vi "AuMT8852B EDR Test Parameter.vi"(0 "VISA session":refnum<visa-resource-name>, 1 "Test (Output power)":T2(ring), 2 "Parameter (Use low frequency)":T1, 3 "Range check? (F)":bool, 4 "Simulate? (F)":bool, 5 "error in (no error)":errorcluster, 6 "Set/Get (Set)":enum16{"Set", "Get"}(ring), 8 "Script (3)":i32=3, 10 "Integer value (0)":i32, 12 "Float value (0)":dbl format="%.3f") -> (11 "Integer value out":i32, 13 "Float value out":dbl format="%.3f", 14 "VISA session out":refnum<visa-resource-name>, 19 "error out":errorcluster)   [LabVIEW 2017]
doc: "Anritsu MT8852B Bluetooth Tester\n\nWrites or reads a single test parameter from the instrument. This VI is a tool for use by higher-level configuration functions. Not all combinations of tests and parameters are valid.\n\nINPUTS\nSet/Get - whether the parameter will be sent to or received from the instrument.\nScript - test script (1-10) containing the test being configured. Scripts 1 and 2 are read-only.\nTest - type of test to be configured.\nParameter - property of the test to be read or written.\nRange check? - whether or not this VI should reject out-of-range values.\nSimulate? - whether or not this VI should skip the instrument I/O.\nInteger value - value to be written (for integer/boolean parameters).\nFloat value - value to be written (for floating-point parameters).\n\nOUTPUTS\nInteger value out - value read from instrument (for integer/boolean parameters).\nFloat value out - value read from instrument (for floating-point parameters)."
uses:
  <instrlib>/aumt8852B/General/Utilities/MT8850 Test Parameters.ctl
  <instrlib>/aumt8852B/General/Utilities/MT8850 Frequency Units.ctl
panel:
  out "Response":string
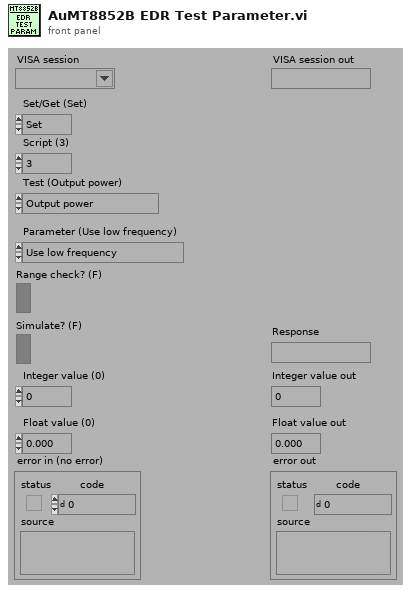
[diagram p1: front panel]
types:
  T1 = typedef "MT8850 Test Parameters.ctl" = enum16{"Use low frequency", "Use medium frequency", "Use high frequency", "Low TX frequency", "Low RX frquency", "Medium TX frequency", "Medium RX frequency", "High TX frequency", "High RX frequency", "Number of packets", "Average high limit", "Average low limit", "Peak power limit", "Max power step limit", "Min power step limit", "f1 average minimum", "f1 average maximum", "f2 maximum", "f1/f2 average maximum", "Hop selection", "Use DH1 packets", "Use DH3 packets", "Use DH5 packets", "1 slot packet drift limit", "3 slot packet drift limit", "5 slot packet drift limit", "Drift rate limit", "TX power level", "Frequency offset", "Symbol timing", "Modulation index", "BER limit", "FER limit", "Use averaging high limit", "Use averaging low limit", "Use peak power limit", "Packet type", "Test control", "Use max power step limit", "Use min power step limit", "Number of cycles", "Use f1 average maximum", "Use f1 average minimum", "Use f2 maximum", "Use f1/f2 average maximum", "Hop mode", "Maximum negative limit", "Maximum positive limit", "Use maximum negative limit", "Use maximum positive limit", "Use 1 slot packet drift limit", "Use 3 slot packet drift limit", "Use 5 slot packet drift limit", "Use drift rate limit", "Use BER limit", "Use FER limit", "Use dirty parameter table", "Use null packet drift limit", "Null packet drift limit", "Minimum power", "Power delay", "Packet count", "Payload toggle", "Output power level", "2DHX packet type", "3DHX packet type", "Number of blocks", "TX and RX low frequency", "TX and RX medium frequency", "TX and RX high frequency", "TX frequency", "RX frequency", "Threshold bit count", "Total test bit count", "Number of bits", "PDPSK to PGFSK lower limit", "PDPSK to PGFSK upper limit", "Initial frequency error upper limit", "Initial frequency error lower limit", "Frequency error upper limit", "Frequency error lower limit", "Block frequency error upper limit", "Block frequency error lower limit", "2Mbs RMS DEVM limit", "3Mbs RMS DEVM limit", "2Mbs Peak DEVM limit", "3Mbs Peak DEVM limit", "2Mbs 99% packets DEVM limit", "3Mbs 99% packets DEVM limit", "Percentage of no error packets limit", "Threshold error limit", "Total test error limit"}
  T2 = enum16{"Output power", "Power control", "Modulation characteristics", "Initial carrier", "Carrier drift", "Single slot sensitivity", "Multiple slot sensitivity", "Maximum input power", "EDR Relative transmit power", "EDR Carrier frequency and stability", "EDR Differential phase encoding", "EDR Sensitivity", "EDR BER floor sensitivity", "EDR Maximum input power"}
  T3 = typedef "MT8850 Frequency Units.ctl" = enum16{"Channel", "Hz", "kHz", "MHz", "GHz"}
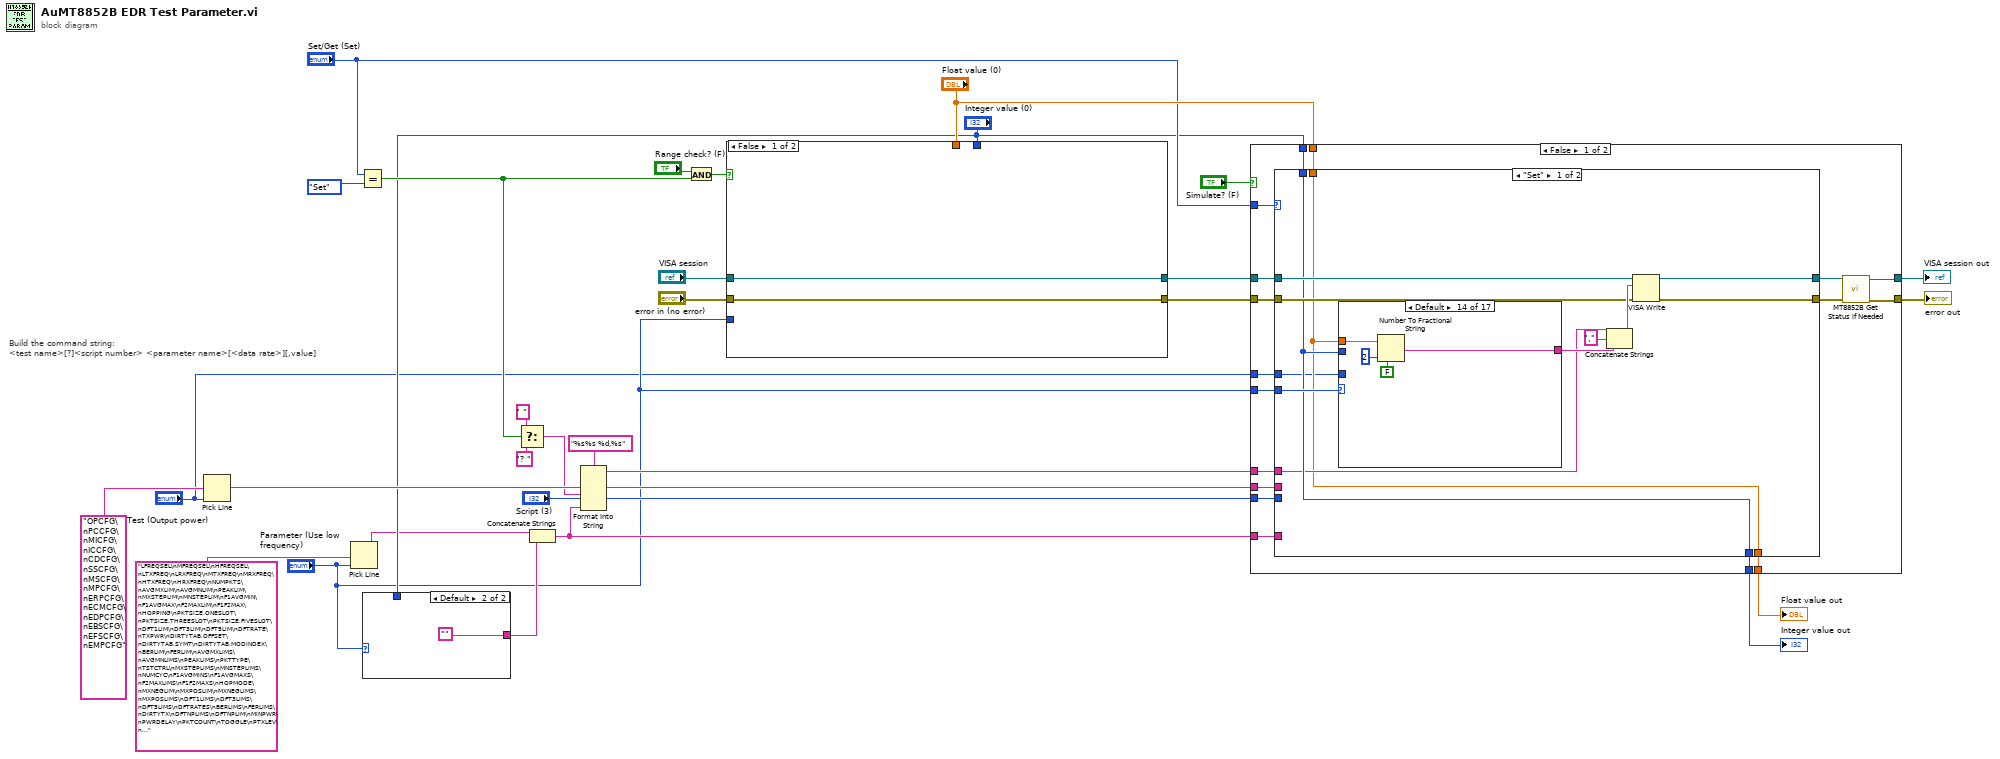
[diagram p0: block diagram]
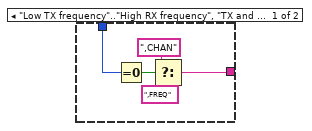
[diagram p2: hidden frame]
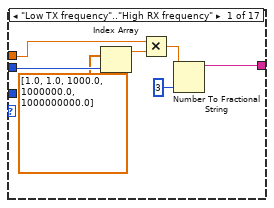
[diagram p3: hidden frame]
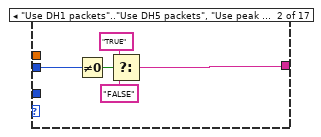
[diagram p4: hidden frame]
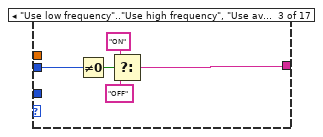
[diagram p5: hidden frame]
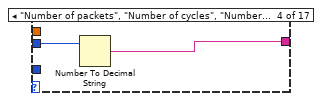
[diagram p6: hidden frame]
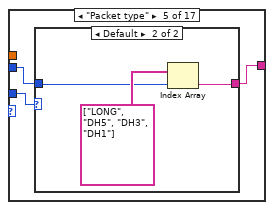
[diagram p7: hidden frame]
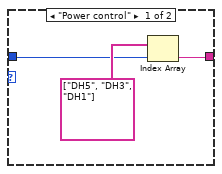
[diagram p8: hidden frame]
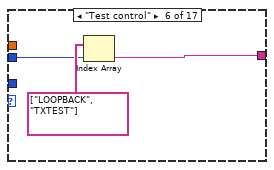
[diagram p9: hidden frame]
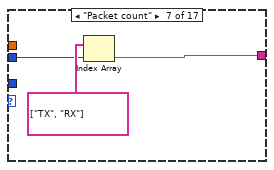
[diagram p10: hidden frame]
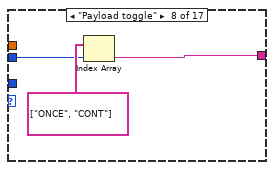
[diagram p11: hidden frame]
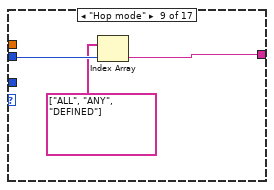
[diagram p12: hidden frame]
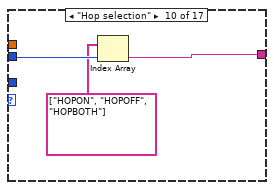
[diagram p13: hidden frame]
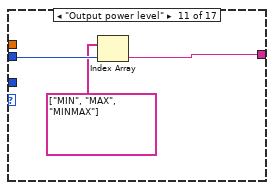
[diagram p14: hidden frame]
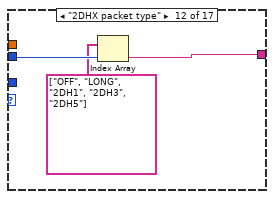
[diagram p15: hidden frame]
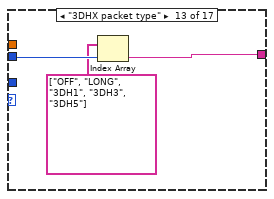
[diagram p16: hidden frame]
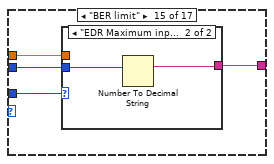
[diagram p17: hidden frame]
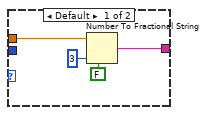
[diagram p18: hidden frame]
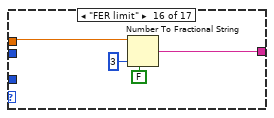
[diagram p19: hidden frame]
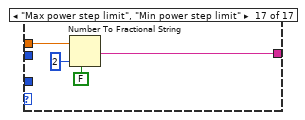
[diagram p20: hidden frame]
diagram:
  # "Build the command string:\n<test name>[?]<script number> <parameter name>[<data rate>][,value]"
  n1 = Pick Line(multi-line string="OPCFG\nPCCFG\nMICFG\nICCFG\nCDCFG\nSSCFG\nMSCFG\nMPCFG\nERPCFG\nECMCFG\nEDPCFG\nEBSCFG\nEFSCFG\nEMPCFG", line index="Test (Output power)") -> (output string=w12:string)  [unwired: 1 in]
  n2 = Pick Line(multi-line string="LFREQSEL\nMFREQSEL\nHFREQSEL\nLTXFREQ\nLRXFREQ\nMTXFREQ\nMRXFREQ\nHTXFREQ\nHRXFREQ\nNUMPKTS\nAVGMXLIM\nAVGMNLIM\nPEAKLIM\nMXSTEPLIM\nMNSTEPLIM\nF1AVGMIN\nF1AVGMAX\nF2MAXLIM\nF1F2MAX\nHOPPING\nPKTSIZE,ONESLOT\nPKTSIZE,THREESLOT\nPKTSIZE,FIVESLOT\nDFT1LIM\nDFT3LIM\nDFT5LIM\nDFTRATE\nTXPWR\nDIRTYTAB,OFFSET\nDIRTYTAB,SYMT\nDIRTYTAB,MODINDEX\nBERLIM\nFERLIM\nAVGMXLIMS\nAVGMNLIMS\nPEAKLIMS\nPKTTYPE\nTSTCTRL\nMXSTEPLIMS\nMNSTEPLIMS\nNUMCYC\nF1AVGMINS\nF1AVGMAXS\nF2MAXLIMS\nF1F2MAXS\nHOPMODE\nMXNEGLIM\nMXPOSLIM\nMXNEGLIMS\nMXPOSLIMS\nDFT1LIMS\nDFT3LIMS\nDFT5LIMS\nDFTRATES\nBERLIMS\nFERLIMS\nDIRTYTX\nDFTNPLIMS\nDFTNPLIM\nMINPWR\nPWRDELAY\nPKTCOUNT\nTOGGLE\nPTXLEV\nDHXPKT,2\nDHXPKT,3\nNUMBLKS\nLFREQ\nMFREQ\nHFREQ\nTXFREQ\nRXFREQ\nTHBITCNT\nTTBITCNT\nNUMBITS\nPDIFFLL\nPDIFFLH\nINITFRQLH\nINITFRQLL\nFREQERLH\nFREQERLL\nBLKFRQLH\nBLKFRQLL\nLRMSDEVM\nHRMSDEVM\nLPKDEVM\nHPKDEVM\nLPCTDEVM\nHPCTDEVM\nPCTPKT\nTHERR\nTTERR\n", line index="Parameter (Use low frequency)") -> (output string=w6:string)  [unwired: 1 in]
  n3 = Equal?(x="Set/Get (Set)", y=enum16{"Set", "Get"}."Set") -> (x = y?=w22:bool)
  n4 = case shown="Default" "Parameter (Use low frequency)" {
    tunnel: "Integer value (0)" -> [w35 _]
    tunnel: [w31 ""] -> w5
    frame "Low TX frequency".."High RX frequency", "TX and RX low frequency".."RX frequency" {
      n5 = Equal To 0?(x=w35) -> (x = 0?=w34:bool)
      n6 = Select(t=",CHAN" ("Substring"), s=w34, f=",FREQ" ("Substring")) -> (s? t:f=w31:string)
    }
    frame Default {
    }
  }
  n7 = Select(t=" ", s=w22, f="? ") -> (s? t:f=w11:string)
  n8 = Concatenate Strings(w6, w5) -> (w7:string)
  n9 = Format Into String(format string="%s%s %d,%s" ("Format String"), w12, w11, "Script (3)", w7) -> (resulting string=w4:string)  [unwired: 2 in, 1 out]
  n10 = And(x="Range check? (F)", y=w22) -> (x .and. y?=w24:bool)
  n11 = case shown="False" w24 {
    tunnel: "Parameter (Use low frequency)" -> [_ w45]
    tunnel: "Integer value (0)" -> [_ w44]
    tunnel: "Float value (0)" -> [_ w43]
    tunnel: "VISA session" -> [w38 w42]
    tunnel: "error in (no error)" -> [w37 w41]
    tunnel: [w38 w40] -> w19
    tunnel: [w37 w39] -> w18
    frame False {
    }
    frame True {
      n12 = case shown="\"Number of packets\", \"Number of cycles\"" w45 {
        tunnel: w44 -> [_ w50 w75 w83 _ _ w105 w111 _ _ _ _ _ _ _ _ _ _]
        tunnel: w43 -> [_ w48 _ _ w92 w100 _ _ w119 w127 w135 w143 w151 w159 w167 w175 w183 w191]
        tunnel: w42 -> [w47 w56 w72 w80 w88 w96 w103 w113 w121 w129 w137 w145 w153 w161 w169 w177 w185 w193]
        tunnel: w41 -> [w46 w55 w71 w79 w87 w95 w104 w112 w120 w128 w136 w144 w152 w160 w168 w176 w184 w192]
        tunnel: [w47 w58 w70 w78 w86 w94 w102 w110 w118 w126 w134 w142 w150 w158 w166 w174 w182 w190] -> w40
        tunnel: [w46 w57 w69 w77 w85 w93 w101 w109 w117 w125 w133 w141 w149 w157 w165 w173 w181 w189] -> w39
        frame Default {
        }
        frame "Low TX frequency".."High RX frequency", "TX and RX low frequency".."RX frequency" {
          n13 = Type Cast(type=MT8850_Frequency_Units."MHz" ("Frequency units (MHz)"), x=w50) -> (*(type *) &x=w51:T3)
          n14 = case shown="\"Channel\"" w51 {
            tunnel: [78.0 2480000000.0 2480000.0 2480.0 2.48] -> w54
            tunnel: [0.0 2402000000.0 2402000.0 2402.0 2.402] -> w53
            frame "Channel" {
            }
            frame "Hz" {
            }
            frame "kHz" {
            }
            frame "MHz" {
            }
            frame "GHz" {
            }
          }
          n15 = call <instrlib>:"AuMT8852B Check Float Range.vi"("Value (0)"=w48, "Check IVI flag first? (T)"=FALSE, "error in (no error)"=w55, "Lower limit (-1)"=w53, "Upper limit (1)"=w54, "VISA session"=w56) -> ("error out"=w57:errorcluster, "VISA session out"=w58:refnum<visa-resource-name>)  [unwired: 4 in]
        }
        frame "Number of packets", "Number of cycles" {
          n16 = call <instrlib>:"AuMT8852B Check Integer Range.vi"("Value (0)"=w75, "Check IVI flag first? (T)"=FALSE, "error in (no error)"=w71, "Lower limit (-1)"=1, "Upper limit (1)"=10000, "VISA session"=w72) -> ("error out"=w69:errorcluster, "VISA session out"=w70:refnum<visa-resource-name>)  [unwired: 4 in]
        }
        frame "Number of blocks" {
          n17 = call <instrlib>:"AuMT8852B Check Integer Range.vi"("Value (0)"=w83, "Check IVI flag first? (T)"=FALSE, "error in (no error)"=w79, "Lower limit (-1)"=1, "Upper limit (1)"=500, "VISA session"=w80) -> ("error out"=w77:errorcluster, "VISA session out"=w78:refnum<visa-resource-name>)  [unwired: 4 in]
        }
        frame "Average high limit".."Peak power limit" {
          n18 = call <instrlib>:"AuMT8852B Check Float Range.vi"("Value (0)"=w92, "Check IVI flag first? (T)"=FALSE, "error in (no error)"=w87, "Lower limit (-1)"=-80.0, "Upper limit (1)"=30.0, "VISA session"=w88) -> ("error out"=w85:errorcluster, "VISA session out"=w86:refnum<visa-resource-name>)  [unwired: 4 in]
        }
        frame "Threshold bit count".."Number of bits" {
          n19 = call <instrlib>:"AuMT8852B Check Float Range.vi"("Value (0)"=w100, "Check IVI flag first? (T)"=FALSE, "error in (no error)"=w95, "Lower limit (-1)"=1.0, "Upper limit (1)"=999.0, "VISA session"=w96) -> ("error out"=w93:errorcluster, "VISA session out"=w94:refnum<visa-resource-name>)  [unwired: 4 in]
        }
        frame "Threshold error limit", "Total test error limit" {
          n20 = call <instrlib>:"AuMT8852B Check Integer Range.vi"("Value (0)"=w105, "Check IVI flag first? (T)"=FALSE, "error in (no error)"=w104, "Lower limit (-1)"=1, "Upper limit (1)"=999, "VISA session"=w103) -> ("error out"=w101:errorcluster, "VISA session out"=w102:refnum<visa-resource-name>)  [unwired: 4 in]
        }
        frame "Max power step limit", "Min power step limit" {
          n21 = call <instrlib>:"AuMT8852B Check Integer Range.vi"("Value (0)"=w111, "Check IVI flag first? (T)"=FALSE, "error in (no error)"=w112, "Lower limit (-1)"=1, "Upper limit (1)"=10, "VISA session"=w113) -> ("error out"=w109:errorcluster, "VISA session out"=w110:refnum<visa-resource-name>)  [unwired: 4 in]
        }
        frame "Frequency offset" {
          n22 = call <instrlib>:"AuMT8852B Check Float Range.vi"("Value (0)"=w119, "Check IVI flag first? (T)"=FALSE, "error in (no error)"=w120, "Lower limit (-1)"=-75000.0, "Upper limit (1)"=75000.0, "VISA session"=w121) -> ("error out"=w117:errorcluster, "VISA session out"=w118:refnum<visa-resource-name>)  [unwired: 4 in]
        }
        frame "Symbol timing" {
          n23 = call <instrlib>:"AuMT8852B Check Float Range.vi"("Value (0)"=w127, "Check IVI flag first? (T)"=FALSE, "error in (no error)"=w128, "Lower limit (-1)"=-20.0, "Upper limit (1)"=20.0, "VISA session"=w129) -> ("error out"=w125:errorcluster, "VISA session out"=w126:refnum<visa-resource-name>)  [unwired: 4 in]
        }
        frame "Modulation index" {
          n24 = call <instrlib>:"AuMT8852B Check Float Range.vi"("Value (0)"=w135, "Check IVI flag first? (T)"=FALSE, "error in (no error)"=w136, "Lower limit (-1)"=0.25, "Upper limit (1)"=0.38, "VISA session"=w137) -> ("error out"=w133:errorcluster, "VISA session out"=w134:refnum<visa-resource-name>)  [unwired: 4 in]
        }
        frame "Minimum power" {
          n25 = call <instrlib>:"AuMT8852B Check Float Range.vi"("Value (0)"=w143, "Check IVI flag first? (T)"=FALSE, "error in (no error)"=w144, "Lower limit (-1)"=-40.0, "Upper limit (1)"=0.0, "VISA session"=w145) -> ("error out"=w141:errorcluster, "VISA session out"=w142:refnum<visa-resource-name>)  [unwired: 4 in]
        }
        frame "Power delay" {
          n26 = call <instrlib>:"AuMT8852B Check Float Range.vi"("Value (0)"=w151, "Check IVI flag first? (T)"=FALSE, "error in (no error)"=w152, "Lower limit (-1)"=0.1, "Upper limit (1)"=100.0, "VISA session"=w153) -> ("error out"=w149:errorcluster, "VISA session out"=w150:refnum<visa-resource-name>)  [unwired: 4 in]
        }
        frame "PDPSK to PGFSK lower limit" {
          n27 = call <instrlib>:"AuMT8852B Check Float Range.vi"("Value (0)"=w159, "Check IVI flag first? (T)"=FALSE, "error in (no error)"=w160, "Lower limit (-1)"=0.0, "Upper limit (1)"=8.0, "VISA session"=w161) -> ("error out"=w157:errorcluster, "VISA session out"=w158:refnum<visa-resource-name>)  [unwired: 4 in]
        }
        frame "PDPSK to PGFSK upper limit" {
          n28 = call <instrlib>:"AuMT8852B Check Float Range.vi"("Value (0)"=w167, "Check IVI flag first? (T)"=FALSE, "error in (no error)"=w168, "Lower limit (-1)"=0.0, "Upper limit (1)"=4.0, "VISA session"=w169) -> ("error out"=w165:errorcluster, "VISA session out"=w166:refnum<visa-resource-name>)  [unwired: 4 in]
        }
        frame "Initial frequency error upper limit".."Block frequency error lower limit" {
          n29 = call <instrlib>:"AuMT8852B Check Float Range.vi"("Value (0)"=w175, "Check IVI flag first? (T)"=FALSE, "error in (no error)"=w176, "Lower limit (-1)"=-100000.0, "Upper limit (1)"=100000.0, "VISA session"=w177) -> ("error out"=w173:errorcluster, "VISA session out"=w174:refnum<visa-resource-name>)  [unwired: 4 in]
        }
        frame "2Mbs RMS DEVM limit".."3Mbs 99% packets DEVM limit" {
          n30 = call <instrlib>:"AuMT8852B Check Float Range.vi"("Value (0)"=w183, "Check IVI flag first? (T)"=FALSE, "error in (no error)"=w184, "Lower limit (-1)"=0.0, "Upper limit (1)"=0.1, "VISA session"=w185) -> ("error out"=w181:errorcluster, "VISA session out"=w182:refnum<visa-resource-name>)  [unwired: 4 in]
        }
        frame "Percentage of no error packets limit" {
          n31 = call <instrlib>:"AuMT8852B Check Float Range.vi"("Value (0)"=w191, "Check IVI flag first? (T)"=FALSE, "error in (no error)"=w192, "Lower limit (-1)"=1.0, "Upper limit (1)"=99.0, "VISA session"=w193) -> ("error out"=w189:errorcluster, "VISA session out"=w190:refnum<visa-resource-name>)  [unwired: 4 in]
        }
      }
    }
  }
  n32 = case shown="False" "Simulate? (F)" {
    tunnel: "Parameter (Use low frequency)" -> [w213 _]
    tunnel: "Integer value (0)" -> [w212 w395]
    tunnel: "Float value (0)" -> [w211 w394]
    tunnel: "Set/Get (Set)" -> [w210 _]
    tunnel: w4 -> [w205 _]
    tunnel: w19 -> [w209 w393]
    tunnel: w18 -> [w208 w392]
    tunnel: [w198 w393] -> w17
    tunnel: [w197 w392] -> w10
    tunnel: [w207 w395] -> w16
    tunnel: [w206 w394] -> w15
    tunnel: w12 -> [w204 _]
    tunnel: w7 -> [w203 _]
    tunnel: "Script (3)" -> [w202 _]
    tunnel: "Test (Output power)" -> [w201 _]
    frame False {
      n33 = case shown="\"Set\"" w210 {
        tunnel: w213 -> [w225 w314]
        tunnel: w212 -> [w217 w311]
        tunnel: w211 -> [w215 w310]
        tunnel: w205 -> [w216 w320]
        tunnel: w209 -> [w221 w322]
        tunnel: w208 -> [w220 w321]
        tunnel: [w219 w316] -> w200
        tunnel: [w218 w315] -> w199
        tunnel: [w217 w313] -> w207
        tunnel: [w215 w312] -> w206
        tunnel: w204 -> [_ w308]
        tunnel: w203 -> [_ w306]
        tunnel: w202 -> [_ w307]
        tunnel: w201 -> [w214 w300]
        frame "Set" {
          n34 = case shown="Default" w225 {
            tunnel: w217 -> [w232 w234 w239 w244 w247 w255 w258 w261 w265 w268 w271 w274 w277 _ w282 _ _]
            tunnel: w215 -> [w230 _ _ _ _ _ _ _ _ _ _ _ _ w281 w284 w293 w299]
            tunnel: [w226 w233 w238 w243 w246 w254 w257 w260 w264 w267 w270 w273 w276 w280 w283 w292 w298] -> w223
            tunnel: w214 -> [_ _ _ _ w245 _ _ _ _ _ _ _ _ _ w285 _ _]
            frame "Low TX frequency".."High RX frequency" {
              n35 = Index Array(array=dbl[] [1.0, 1.0, 1000.0, 1000000.0, 1000000000.0] ("Array Constant"), index=w232) -> (element=w231:dbl)
              n36 = Multiply(x=w230, y=w231) -> (x*y=w228:dbl)
              n37 = Number To Fractional String(number=w228, precision (6)=i16 3) -> (F-format string=w226:string)  [unwired: 2 in]
            }
            frame "Use DH1 packets".."Use DH5 packets", "Use peak power limit", "Use max power step limit", "Use min power step limit", "Use f1 average maximum".."Use f1/f2 average maximum", "Use maximum negative limit".."Use FER limit" {
              n38 = Not Equal To 0?(x=w234) -> (x != 0?=w237:bool)
              n39 = Select(t="TRUE", s=w237, f="FALSE") -> (s? t:f=w233:string)
            }
            frame "Use low frequency".."Use high frequency", "Use averaging high limit", "Use averaging low limit", "Use dirty parameter table", "Use null packet drift limit" {
              n40 = Not Equal To 0?(x=w239) -> (x != 0?=w242:bool)
              n41 = Select(t="ON", s=w242, f="OFF") -> (s? t:f=w238:string)
            }
            frame "Number of packets", "Number of cycles", "Number of blocks", "Threshold error limit", "Total test error limit" {
              n42 = Number To Decimal String(number=w244) -> (decimal integer string=w243:string)  [unwired: 1 in]
            }
            frame "Packet type" {
              n43 = case shown="Default" w245 {
                tunnel: w247 -> [w249 w252]
                tunnel: [w248 w251] -> w246
                frame "Power control" {
                  n44 = Index Array(array=string[] ["DH5", "DH3", "DH1"] ("Array Constant"), index=w249) -> (element=w248:string)
                }
                frame Default {
                  n45 = Index Array(array=string[] ["LONG", "DH5", "DH3", "DH1"] ("Array Constant"), index=w252) -> (element=w251:string)
                }
              }
            }
            frame "Test control" {
              n46 = Index Array(array=string[] ["LOOPBACK", "TXTEST"] ("Array Constant"), index=w255) -> (element=w254:string)
            }
            frame "Packet count" {
              n47 = Index Array(array=string[] ["TX", "RX"] ("Array Constant"), index=w258) -> (element=w257:string)
            }
            frame "Payload toggle" {
              n48 = Index Array(array=string[] ["ONCE", "CONT"] ("Array Constant"), index=w261) -> (element=w260:string)
            }
            frame "Hop mode" {
              n49 = Index Array(array=string[] ["ALL", "ANY", "DEFINED"] ("Array Constant"), index=w265) -> (element=w264:string)
            }
            frame "Hop selection" {
              n50 = Index Array(array=string[] ["HOPON", "HOPOFF", "HOPBOTH"] ("Array Constant"), index=w268) -> (element=w267:string)
            }
            frame "Output power level" {
              n51 = Index Array(array=string[] ["MIN", "MAX", "MINMAX"] ("Array Constant"), index=w271) -> (element=w270:string)
            }
            frame "2DHX packet type" {
              n52 = Index Array(array=string[] ["OFF", "LONG", "2DH1", "2DH3", "2DH5"] ("Array Constant"), index=w274) -> (element=w273:string)
            }
            frame "3DHX packet type" {
              n53 = Index Array(array=string[] ["OFF", "LONG", "3DH1", "3DH3", "3DH5"] ("Array Constant"), index=w277) -> (element=w276:string)
            }
            frame Default {
              n54 = Number To Fractional String(use system decimal point (T)=FALSE, number=w281, precision (6)=i16 2) -> (F-format string=w280:string)  [unwired: 1 in]
            }
            frame "BER limit" {
              n55 = case shown="\"EDR Maximum input power\"" w285 {
                tunnel: w284 -> [w287 _]
                tunnel: [w286 w291] -> w283
                tunnel: w282 -> [_ w290]
                frame Default {
                  n56 = Number To Fractional String(use system decimal point (T)=FALSE, number=w287, precision (6)=i16 3) -> (F-format string=w286:string)  [unwired: 1 in]
                }
                frame "EDR Maximum input power" {
                  n57 = Number To Decimal String(number=w290) -> (decimal integer string=w291:string)  [unwired: 1 in]
                }
              }
            }
            frame "FER limit" {
              n58 = Number To Fractional String(use system decimal point (T)=FALSE, number=w293, precision (6)=i16 3) -> (F-format string=w292:string)  [unwired: 1 in]
            }
            frame "Max power step limit", "Min power step limit" {
              n59 = Number To Fractional String(use system decimal point (T)=FALSE, number=w299, precision (6)=i16 2) -> (F-format string=w298:string)  [unwired: 1 in]
            }
          }
          n60 = Concatenate Strings(w216, "," ("Substring"), w223) -> (w222:string)
          n61 = VISA Write(VISA resource name=w221, write buffer=w222, error in (no error)=w220) -> (VISA resource name out=w219:refnum<visa-resource-name>, error out=w218:errorcluster)  [unwired: 1 out]
        }
        frame "Get" {
          n62 = VISA Write(VISA resource name=w322, write buffer=w320, error in (no error)=w321) -> (VISA resource name out=w319:refnum<visa-resource-name>, error out=w318:errorcluster)  [unwired: 1 out]
          n63 = Format Into String(format string="%s %d,%s,%%s" ("Format String"), w308, w307, w306) -> (resulting string=w305:string)  [unwired: 2 in, 1 out]
          n64 = VISA Read(VISA resource name=w319, byte count=u32 100 ("byte count (0)"), error in (no error)=w318) -> (VISA resource name out=w316:refnum<visa-resource-name>, read buffer=w303:string, error out=w315:errorcluster)  [unwired: 1 out]
          n65 = Match Pattern(string=w303, regular expression="\n$") -> (before substring=w301:string)  [unwired: 1 in, 3 out]
          n66 = Scan From String(format string=w305, input string=w301) -> (output 1=w304:string)  [unwired: 3 in, 3 out]
          "Response" <- w304
          n67 = case shown="\"Number of packets\", \"Number of cycles\", \"Number of blocks\", \"Threshold error limit\", \"Total test error limit\"" w314 {
            tunnel: w304 -> [w328 w331 w334 w338 w342 w346 w350 w354 w358 w362 w366 w370 w375 w385 w391]
            tunnel: [w327 w330 w333 w337 w341 w345 w349 w353 w357 w361 w365 w368 w373 w383 w386] -> w313
            tunnel: [w326 w329 w332 w336 w340 w344 w348 w352 w356 w360 w364 w369 w374 w384 w387] -> w312
            tunnel: w311 -> [_ _ _ _ _ _ _ _ _ _ _ w368 w372 w383 w386]
            tunnel: w310 -> [w326 w329 w332 w336 w340 w344 w348 w352 w356 w360 w364 _ w371 _ _]
            tunnel: w300 -> [_ _ _ _ _ _ _ _ _ _ _ _ w376 _ _]
            frame "Use low frequency".."Use high frequency", "Use DH1 packets".."Use DH5 packets", "Use averaging high limit".."Use peak power limit", "Use max power step limit", "Use min power step limit", "Use f1 average maximum".."Use f1/f2 average maximum", "Use maximum negative limit".."Use null packet drift limit" {
              n68 = Equal?(x=w328, y=string[] ["TRUE", "ON"] ("Array Constant")) -> (x = y?=w324:bool[])
              n69 = Or Array Elements(Boolean array=w324) -> (logical OR=w323:bool)
              n70 = Boolean To (0,1)(Boolean=w323) -> (0, 1=w327:i16)
            }
            frame "Number of packets", "Number of cycles", "Number of blocks", "Threshold error limit", "Total test error limit" {
              n71 = Decimal String To Number(string=w331) -> (number=w330:i32)  [unwired: 2 in, 1 out]
            }
            frame "Packet type" {
              n72 = Match First String(2:string[] ["LONG", "DH5", "DH3", "DH1"] ("Array Constant"), 3:w334) -> (0:w333:i32)  [unwired: 1 out]
            }
            frame "Test control" {
              n73 = Match First String(2:string[] ["LOOPBACK", "TXTEST"] ("Array Constant"), 3:w338) -> (0:w337:i32)  [unwired: 1 out]
            }
            frame "Packet count" {
              n74 = Match First String(2:string[] ["TX", "RX"] ("Array Constant"), 3:w342) -> (0:w341:i32)  [unwired: 1 out]
            }
            frame "Payload toggle" {
              n75 = Match First String(2:string[] ["ONCE", "CONT"] ("Array Constant"), 3:w346) -> (0:w345:i32)  [unwired: 1 out]
            }
            frame "Hop mode" {
              n76 = Match First String(2:string[] ["ALL", "ANY", "DEFINED"] ("Array Constant"), 3:w350) -> (0:w349:i32)  [unwired: 1 out]
            }
            frame "Hop selection" {
              n77 = Match First String(2:string[] ["HOPON", "HOPOFF", "HOPBOTH"] ("Array Constant"), 3:w354) -> (0:w353:i32)  [unwired: 1 out]
            }
            frame "Output power level" {
              n78 = Match First String(2:string[] ["MIN", "MAX", "MINMAX"] ("Array Constant"), 3:w358) -> (0:w357:i32)  [unwired: 1 out]
            }
            frame "2DHX packet type" {
              n79 = Match First String(2:string[] ["OFF", "LONG", "2DH1", "2DH3", "2DH5"] ("Array Constant"), 3:w362) -> (0:w361:i32)  [unwired: 1 out]
            }
            frame "3DHX packet type" {
              n80 = Match First String(2:string[] ["OFF", "LONG", "3DH1", "3DH3", "3DH5"] ("Array Constant"), 3:w366) -> (0:w365:i32)  [unwired: 1 out]
            }
            frame Default {
              n81 = Fract/Exp String To Number(string=w370) -> (number=w369:dbl)  [unwired: 3 in, 1 out]
            }
            frame "BER limit" {
              n82 = case shown="Default" w376 {
                tunnel: w375 -> [w379 w382]
                tunnel: [w378 w380] -> w374
                tunnel: [w377 w381] -> w373
                tunnel: w372 -> [w377 _]
                tunnel: w371 -> [_ w380]
                frame Default {
                  n83 = Fract/Exp String To Number(string=w379) -> (number=w378:dbl)  [unwired: 3 in, 1 out]
                }
                frame "EDR Maximum input power" {
                  n84 = Decimal String To Number(string=w382) -> (number=w381:i32)  [unwired: 2 in, 1 out]
                }
              }
            }
            frame "Max power step limit", "Min power step limit" {
              n85 = Fract/Exp String To Number(string=w385) -> (number=w384:dbl)  [unwired: 3 in, 1 out]
            }
            frame "Low TX frequency".."High RX frequency" {
              n86 = Fract/Exp String To Number(string=w391) -> (number=w389:dbl)  [unwired: 3 in, 1 out]
              n87 = Index Array(array=dbl[] [1.0, 1.0, 1000.0, 1000000.0, 1000000000.0] ("Array Constant"), index=w386) -> (element=w388:dbl)
              n88 = Divide(x=w389, y=w388) -> (x/y=w387:dbl)
            }
          }
        }
      }
      n89 = call <instrlib>:"MT8852B Get Status if Needed.vi"("error in (no error)"=w199, "VISA session"=w200) -> ("error out"=w197:errorcluster, "VISA session out"=w198:refnum<visa-resource-name>)  [unwired: 8 in]
    }
    frame True {
    }
  }
  "VISA session out" <- w17
  "error out" <- w10
  "Integer value out" <- w16
  "Float value out" <- w15
